vi "compareDataGcodeFile.vi"(8 "error in (no error)":errorcluster, 11 "ParameterConf in":refnum<class "ParameterConf.lvclass">) -> (0 "error out":errorcluster, 3 "ParameterConf out":refnum<class "ParameterConf.lvclass">)   [LabVIEW 2017, in "LibraryGcode.lvlib" / "ParameterConf.lvclass"]
uses:
  ParameterConf.lvclass
panel:
  in  "Boolean":bool
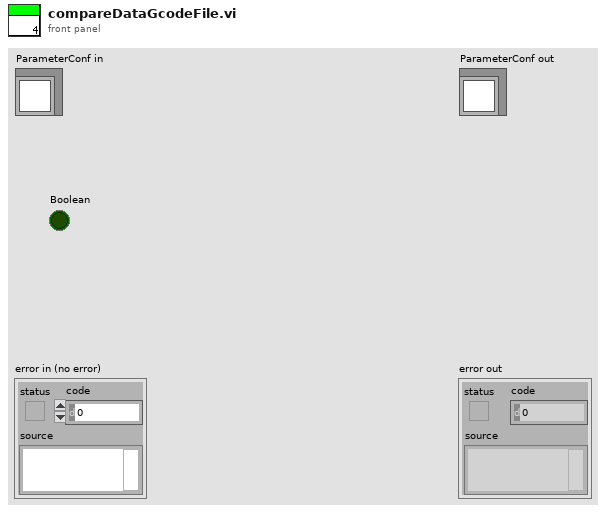
[diagram p1: front panel]
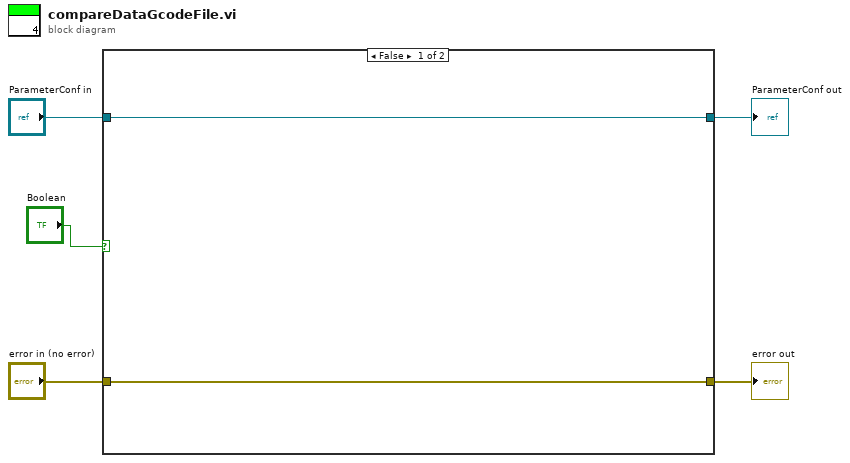
[diagram p0: block diagram]
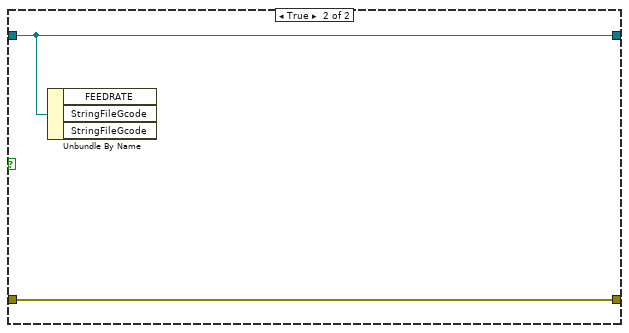
[diagram p2: hidden frame]
diagram:
  n1 = case shown="False" "Boolean" {
    tunnel: [w7 w8] -> w4
    tunnel: "ParameterConf in" -> [w7 w8]
    tunnel: [w6 w9] -> w1
    tunnel: "error in (no error)" -> [w6 w9]
    frame False {
    }
    frame True {
      n2 = Unbundle By Name(w8) -> ()  [unwired: 3 out]
    }
  }
  "error out" <- w1
  "ParameterConf out" <- w4
